vi "CAN.vi"() -> ()   [LabVIEW 2020]
uses:
  Global_Variable/Global.vi
  Other/ZLG_CAN/ZLG_CAN.lvlib
panel:
  in  "CAN 通道":u32(ring) items=["0", "1"]
  in  "索引":u32(ring) items=["0", "1", "2", "3", "4", "5", "6", "7", "8"]
  in  "设备类型":u32(ring)=27 items=["PCI5121"=1, "PCI9810"=2, "USBCAN1"=3, "USBCAN2"=4, "PCI9820"=5, "PCI5110"=7, "PC104CAN"=11, "CANETUDP"=12, "PCI9840B"=14, "PC104C2"=15, "PCI9820I"=16, "CANETTCP"=17, "PCIE9221"=24, "PCI5010U"=19, "USBCAN_E_U"=20, "USBCAN_2E_U"=21, "PCI5020U"=22, "PCIE9120I"=27, "PCIE9110I"=28, "PCIE9140I"=29]
  in  "Stop":bool
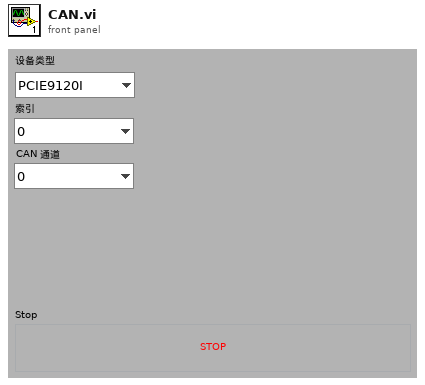
[diagram p1: front panel]
types:
  T1 = cluster{"波特率":u32, "ID":u32, "帧类型":enum8{"标准帧", "扩展帧"}, "帧格式":enum16{"数据帧", "远程帧"}, "周期(ms)":u32}
  T2 = typedef "ZLG_CAN.lvlib/Start_CAN (Reply Payload)--cluster.ctl" = cluster{"Success":bool, "Start_CAN_error":errorcluster}
  T3 = cluster{u8, u8, "y":u8, "y":u8, "y":u8, "y":u8, "y":u8, "y":u8}
  T4 = cluster{"y":u8, "y":u8, "y":u8, u8, u8, "y":u8, "y":u8, "y":u8}
  T5 = cluster{"[0]":u8, "[1]":u8, "[2]":u8, "[3]":u8, "[4]":u8, "[5]":u8, "[6]":u8, "[7]":u8}
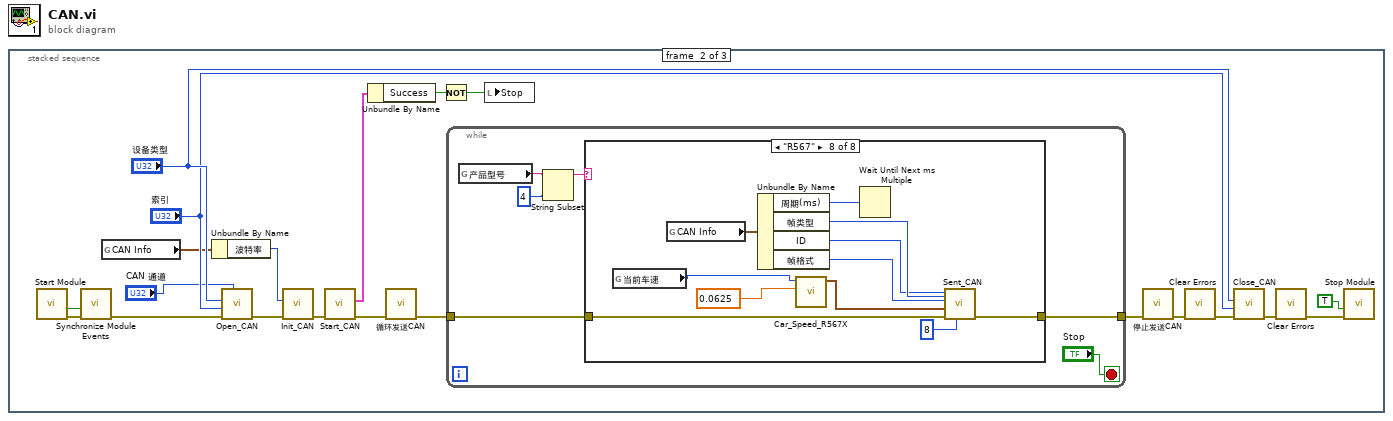
[diagram p0: block diagram]
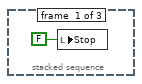
[diagram p2: hidden frame]
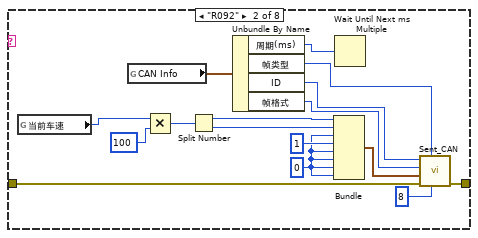
[diagram p4: hidden frame]
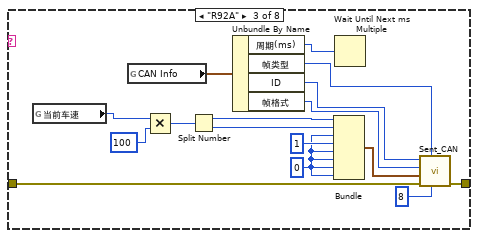
[diagram p5: hidden frame]
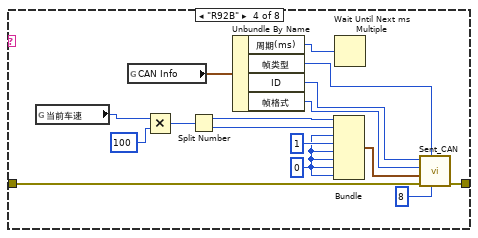
[diagram p6: hidden frame]
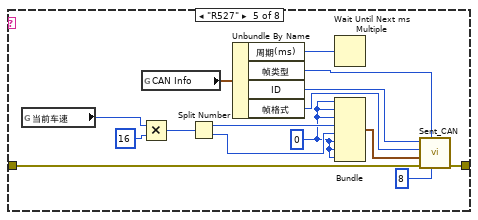
[diagram p7: hidden frame]
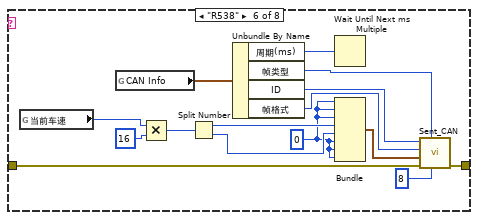
[diagram p8: hidden frame]
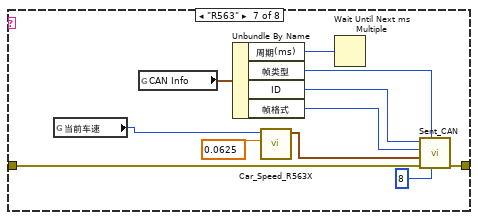
[diagram p9: hidden frame]
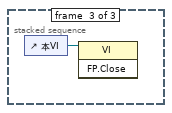
[diagram p10: hidden frame]
diagram:
  n1 = stacked-sequence {
    frame #0 {
      n2 = local write "Stop"(FALSE ("Stop")) -> ()
    }
    frame #1 {
      n3 = call "Start Module.vi"() -> ("error out"=w22:errorcluster, "Wait for Event Sync?"=w21:bool)  [unwired: 8 in, 2 out]
      n4 = call "Synchronize Module Events.vi"("error in (no error)"=w22, "Wait for Event Sync?"=w21) -> ("error out"=w20:errorcluster)  [unwired: 9 in]
      n5 = global read "Global.vi" "CAN Info"() -> (w7:T1)
      n6 = Unbundle By Name(w7) -> ("波特率"=w12:u32)
      n7 = call "Open_CAN.vi"("CAN 通道"="CAN 通道", "error in (no error)"=w20, "索引"="索引", "设备类型"="设备类型") -> ("error out"=w17:errorcluster)  [unwired: 7 in]
      n8 = call "Init_CAN.vi"("error in (no error)"=w17, "波特率"=w12) -> ("error out"=w13:errorcluster)  [unwired: 9 in]
      n9 = call "Start_CAN.vi"("error in (no error)"=w13) -> ("error out"=w6:errorcluster, "Reply Payload"=w15:T2)  [unwired: 8 in, 1 out]
      n10 = Unbundle By Name(w15) -> ("Success"=w14:bool)
      n11 = call "循环发送CAN.vi"("错误输入"=w6) -> ("错误输出"=w5:errorcluster)  [unwired: 10 in]
      n12 = Not(x=w14) -> (.not. x?=w2:bool)
      n13 = while {
        tunnel: w5 -> [w28]
        tunnel: [w27] -> w4
        stop <- "Stop" stop-if-true
        n14 = global read "Global.vi" "产品型号"() -> (w25:string)
        n15 = String Subset(string=w25, length (rest)=4 ("长度（剩余）")) -> (substring=w23:string)  [unwired: 1 in]
        n16 = case shown="\"R567\"" w23 {
          tunnel: w28 -> [w29 w45 w61 w77 w92 w107 w118 w129]
          tunnel: [w29 w44 w60 w76 w91 w106 w117 w128] -> w27
          frame "假", Default {
          }
          frame "R092" {
            w31 = u8 0 ("y")
            n17 = global read "Global.vi" "当前车速"() -> (w30:u16)
            n18 = global read "Global.vi" "CAN Info"() -> (w32:T1)
            n19 = Multiply(x=w30, y=u16 100) -> (x*y=w42:u16)
            n20 = Split Number(x=w42) -> (hi(x)=w41:u8, lo(x)=w40:u8)
            n21 = Unbundle By Name(w32) -> ("周期(ms)"=w36:u32, "帧类型"=w34:enum8{"标准帧", "扩展帧"}, "ID"=w33:u32, "帧格式"=w35:enum16{"数据帧", "远程帧"})
            n22 = Bundle(w41, w40, "y"=w31, "y"=u8 1, "y"=w31, "y"=w31, "y"=w31, "y"=w31) -> (w38:T3)  [unwired: 1 in]
            n23 = Wait Until Next ms Multiple(millisecond multiple=w36) -> ()  [unwired: 1 out]
            n24 = call "Sent_CAN.vi"("帧长度"=u8 8, "帧类型"=w34, "error in (no error)"=w45, "帧数据"=w38, "帧格式"=w35, "ID"=w33) -> ("error out"=w44:errorcluster)  [unwired: 5 in]
          }
          frame "R92A" {
            w47 = u8 0 ("y")
            n25 = global read "Global.vi" "当前车速"() -> (w46:u16)
            n26 = global read "Global.vi" "CAN Info"() -> (w48:T1)
            n27 = Multiply(x=w46, y=u16 100) -> (x*y=w58:u16)
            n28 = Split Number(x=w58) -> (hi(x)=w57:u8, lo(x)=w56:u8)
            n29 = Unbundle By Name(w48) -> ("周期(ms)"=w52:u32, "帧类型"=w50:enum8{"标准帧", "扩展帧"}, "ID"=w49:u32, "帧格式"=w51:enum16{"数据帧", "远程帧"})
            n30 = Bundle(w57, w56, "y"=w47, "y"=u8 1, "y"=w47, "y"=w47, "y"=w47, "y"=w47) -> (w54:T3)  [unwired: 1 in]
            n31 = Wait Until Next ms Multiple(millisecond multiple=w52) -> ()  [unwired: 1 out]
            n32 = call "Sent_CAN.vi"("帧长度"=u8 8, "帧类型"=w50, "error in (no error)"=w61, "帧数据"=w54, "帧格式"=w51, "ID"=w49) -> ("error out"=w60:errorcluster)  [unwired: 5 in]
          }
          frame "R92B" {
            w63 = u8 0 ("y")
            n33 = global read "Global.vi" "当前车速"() -> (w62:u16)
            n34 = global read "Global.vi" "CAN Info"() -> (w64:T1)
            n35 = Multiply(x=w62, y=u16 100) -> (x*y=w74:u16)
            n36 = Split Number(x=w74) -> (hi(x)=w73:u8, lo(x)=w72:u8)
            n37 = Unbundle By Name(w64) -> ("周期(ms)"=w68:u32, "帧类型"=w66:enum8{"标准帧", "扩展帧"}, "ID"=w65:u32, "帧格式"=w67:enum16{"数据帧", "远程帧"})
            n38 = Bundle(w73, w72, "y"=w63, "y"=u8 1, "y"=w63, "y"=w63, "y"=w63, "y"=w63) -> (w70:T3)  [unwired: 1 in]
            n39 = Wait Until Next ms Multiple(millisecond multiple=w68) -> ()  [unwired: 1 out]
            n40 = call "Sent_CAN.vi"("帧长度"=u8 8, "帧类型"=w66, "error in (no error)"=w77, "帧数据"=w70, "帧格式"=w67, "ID"=w65) -> ("error out"=w76:errorcluster)  [unwired: 5 in]
          }
          frame "R527" {
            w79 = u8 0 ("y")
            n41 = global read "Global.vi" "当前车速"() -> (w78:u16)
            n42 = Multiply(x=w78, y=u16 16) -> (x*y=w89:u16)
            n43 = global read "Global.vi" "CAN Info"() -> (w82:T1)
            n44 = Split Number(x=w89) -> (hi(x)=w81:u8, lo(x)=w80:u8)
            n45 = Unbundle By Name(w82) -> ("周期(ms)"=w86:u32, "帧类型"=w84:enum8{"标准帧", "扩展帧"}, "ID"=w83:u32, "帧格式"=w85:enum16{"数据帧", "远程帧"})
            n46 = Wait Until Next ms Multiple(millisecond multiple=w86) -> ()  [unwired: 1 out]
            n47 = Bundle("y"=w79, "y"=w79, "y"=w79, w81, w80, "y"=w79, "y"=w79, "y"=w79) -> (w88:T4)  [unwired: 1 in]
            n48 = call "Sent_CAN.vi"("帧长度"=u8 8, "帧类型"=w84, "error in (no error)"=w92, "帧数据"=w88, "帧格式"=w85, "ID"=w83) -> ("error out"=w91:errorcluster)  [unwired: 5 in]
          }
          frame "R538" {
            w94 = u8 0 ("y")
            n49 = global read "Global.vi" "当前车速"() -> (w93:u16)
            n50 = global read "Global.vi" "CAN Info"() -> (w97:T1)
            n51 = Multiply(x=w93, y=u16 16) -> (x*y=w104:u16)
            n52 = Split Number(x=w104) -> (hi(x)=w96:u8, lo(x)=w95:u8)
            n53 = Unbundle By Name(w97) -> ("周期(ms)"=w101:u32, "帧类型"=w99:enum8{"标准帧", "扩展帧"}, "ID"=w98:u32, "帧格式"=w100:enum16{"数据帧", "远程帧"})
            n54 = Wait Until Next ms Multiple(millisecond multiple=w101) -> ()  [unwired: 1 out]
            n55 = Bundle("y"=w94, "y"=w94, "y"=w94, w96, w95, "y"=w94, "y"=w94, "y"=w94) -> (w103:T4)  [unwired: 1 in]
            n56 = call "Sent_CAN.vi"("帧长度"=u8 8, "帧类型"=w99, "error in (no error)"=w107, "帧数据"=w103, "帧格式"=w100, "ID"=w98) -> ("error out"=w106:errorcluster)  [unwired: 5 in]
          }
          frame "R563" {
            n57 = global read "Global.vi" "当前车速"() -> (w108:u16)
            n58 = global read "Global.vi" "CAN Info"() -> (w111:T1)
            n59 = Unbundle By Name(w111) -> ("周期(ms)"=w115:u32, "帧类型"=w113:enum8{"标准帧", "扩展帧"}, "ID"=w112:u32, "帧格式"=w114:enum16{"数据帧", "远程帧"})
            n60 = call "Car_Speed_R563X.vi"("精度"=0.0625, "车速"=w108) -> ("报文"=w109:T5)  [unwired: 9 in]
            n61 = Wait Until Next ms Multiple(millisecond multiple=w115) -> ()  [unwired: 1 out]
            n62 = call "Sent_CAN.vi"("帧长度"=u8 8, "帧类型"=w113, "error in (no error)"=w118, "帧数据"=w109, "帧格式"=w114, "ID"=w112) -> ("error out"=w117:errorcluster)  [unwired: 5 in]
          }
          frame "R567" {
            n63 = global read "Global.vi" "当前车速"() -> (w119:u16)
            n64 = global read "Global.vi" "CAN Info"() -> (w122:T1)
            n65 = Unbundle By Name(w122) -> ("周期(ms)"=w126:u32, "帧类型"=w124:enum8{"标准帧", "扩展帧"}, "ID"=w123:u32, "帧格式"=w125:enum16{"数据帧", "远程帧"})
            n66 = call "Car_Speed_R567X.vi"("精度"=0.0625, "车速"=w119) -> ("报文"=w121:T5)  [unwired: 9 in]
            n67 = Wait Until Next ms Multiple(millisecond multiple=w126) -> ()  [unwired: 1 out]
            n68 = call "Sent_CAN.vi"("帧长度"=u8 8, "帧类型"=w124, "error in (no error)"=w129, "帧数据"=w121, "帧格式"=w125, "ID"=w123) -> ("error out"=w128:errorcluster)  [unwired: 5 in]
          }
        }
      }
      n69 = local write "Stop"(w2) -> ()
      n70 = call "停止发送CAN.vi"("错误输入"=w4) -> ("错误输出"=w3:errorcluster)  [unwired: 10 in]
      n71 = call <vilib>:"Clear Errors.vi"("error in (no error)"=w3) -> ("error out"=w8:errorcluster)  [unwired: 5 in, 1 out]
      n72 = call "Close_CAN.vi"("error in (no error)"=w8, "索引"="索引", "设备类型"="设备类型") -> ("error out"=w11:errorcluster)  [unwired: 8 in]
      n73 = call <vilib>:"Clear Errors.vi"("error in (no error)"=w11) -> ("error out"=w9:errorcluster)  [unwired: 5 in, 1 out]
      n74 = call "Stop Module.vi"("error in (no error)"=w9, "Wait for Module to Stop? (F)"=TRUE) -> ()  [unwired: 9 in, 1 out]
    }
    frame #2 {
      n75 = control-ref of="本VI"() -> (w130:refnum<vi>)
      n76 = invoke class="VI" method="FP.Close"(reference=w130) -> ()  [unwired: 2 in, 3 out]
    }
  }
